vi "Process Data.vi"(6 "dt":dbl, 8 "error in (no error)":errorcluster, 9 "t0":dbl, 10 "Data":dbl[][](array[numeric]), 11 "DataProcessor in":refnum<class "DataProcessor.lvclass">) -> (0 "error out":errorcluster, 3 "DataProcessor out":refnum<class "DataProcessor.lvclass">)   [LabVIEW 2020, in "Volatus.lvlib" / "DataProcessor.lvclass"]
uses:
  DataProcessor.lvclass
  C:/dev/lv20CE/relink/lv-volatus/Volatus/Task/Task.lvclass
  DataProcessor.lvclass/DataProcessor.ctl
  DataHandlerAPI/DataHandlerAPI.lvclass/DataHandlerAPI.ctl
  DataHandler Messages/New Data Msg/New Data Msg.lvclass/New Data Msg.ctl
  <vilib>/ActorFramework/Message Enqueuer/Message Enqueuer.lvclass/Message Enqueuer.ctl
  Task/Task.lvclass/Task.ctl
  TelemetryAPI/TelemetryAPI.lvclass/TelemetryAPI.ctl
  Polynomial Evaluate.vi
  DataHandlerAPI/New Data.vi
  <vilib>/Analysis/baseanly.llb/Mean.vi
  <vilib>/Analysis/baseanly.llb/Mean (DBL).vi
  Task/Publish Group.vi
  Polynomial Remove Trailing Zeros.vi
  DataHandler Messages/New Data Msg/Send New Data.vi
  TelemetryAPI/Publish Group.vi
  <vilib>/ActorFramework/Message Enqueuer/Enqueue.vi
  DataHandler Messages/New Data Msg/New Data Msg.lvclass
  C:/Program Files (x86)/National Instruments/LabVIEW 2020/vi.lib/ActorFramework/Message/Message.lvclass
  lv-vecto/Vecto/Group/Group.lvclass
  C:/dev/lv20CE/relink/lv-vecto/Vecto/GroupAbstract/GroupAbstract.lvclass
  <vilib>/ActorFramework/Message Priority Queue/Priority Enqueue.vi
  lv-vecto/Vecto/Group/Update Values.vi
  lv-vecto/Vecto/RemoteDataService/Publish Group.vi
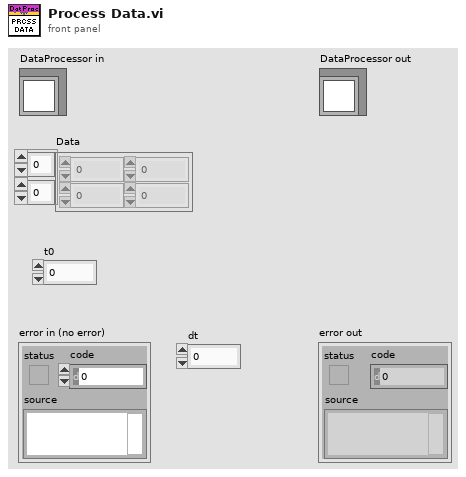
[diagram p1: front panel]
types:
  T1 = typedef "Volatus.lvlib/Processing Type.ctl" = enum16{"Scaling", "Redlines", "Logger"}
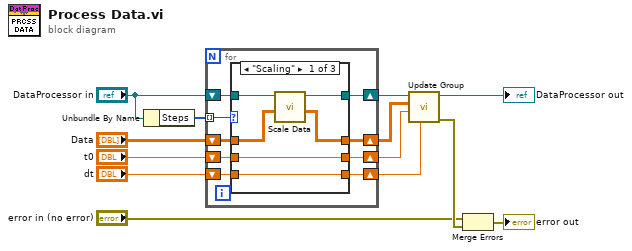
[diagram p0: block diagram]
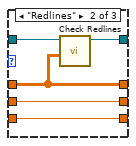
[diagram p2: hidden frame]
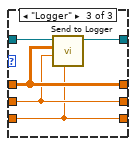
[diagram p3: hidden frame]
diagram:
  n1 = Unbundle By Name("DataProcessor in") -> ("Steps"=w13:T1[])
  n2 = for {
    tunnel: w13 -> [w14] mode=indexing
    shift-right: [w17] -> w6
    shift-left: "Data" -> [w22]
    shift-right: [w21] -> w5
    shift-left: "t0" -> [w20]
    shift-right: [w19] -> w4
    shift-left: "dt" -> [w18]
    shift-right: [w15] -> w8
    shift-left: "DataProcessor in" -> [w16]
    n3 = case shown="\"Scaling\"" w14 {
      tunnel: w22 -> [w26 w29 w37]
      tunnel: [w28 w33 w36] -> w21
      tunnel: w20 -> [w28 w33 w36]
      tunnel: [w27 w32 w35] -> w19
      tunnel: w18 -> [w27 w32 w35]
      tunnel: [w25 w29 w37] -> w17
      tunnel: w16 -> [w24 w31 w38]
      tunnel: [w23 w30 w34] -> w15
      frame "Scaling" {
        n4 = call "Scale Data.vi"("Data"=w26, "DataProcessor in"=w24) -> ("Scaled Data"=w25:dbl[][], "DataProcessor out"=w23:refnum<class "DataProcessor.lvclass">)  [unwired: 8 in]
      }
      frame "Redlines" {
        n5 = call "Check Redlines.vi"("Data"=w29, "DataProcessor in"=w31) -> ("DataProcessor out"=w30:refnum<class "DataProcessor.lvclass">)  [unwired: 8 in, 1 out]
      }
      frame "Logger" {
        n6 = call "Send to Logger.vi"("dt"=w35, "t0"=w36, "Data"=w37, "DataProcessor in"=w38) -> ("DataProcessor out"=w34:refnum<class "DataProcessor.lvclass">)  [unwired: 6 in, 1 out]
      }
    }
  }
  n7 = call "Update Group.vi"("dt"=w4, "t0"=w5, "Data"=w6, "DataProcessor in"=w8) -> ("error out"=w3:errorcluster, "DataProcessor out"=→"DataProcessor out":refnum<class "DataProcessor.lvclass">)  [unwired: 6 in]
  n8 = Merge Errors("error in (no error)", w3) -> (→"error out":errorcluster)
